vi "Unsubscribe.vi"(8 "error in (no error)":errorcluster, 10 "Message In":refnum<class "Message.lvclass">, 11 "System Actor in":refnum<class "System Actor.lvclass">) -> (0 "error out":errorcluster, 3 "System Actor out":refnum<class "System Actor.lvclass">)   [LabVIEW 2019, in "System Actor.lvclass"]
uses:
  System Actor.lvclass
  Message/Message.lvclass
  Message/Message.lvclass/Message.ctl
  System Actor.lvclass/System Actor.ctl
  Message/Public Data/Read Subscriber.vi
  Subscriber/Subscriber.lvclass
  Observer/Observer.lvclass
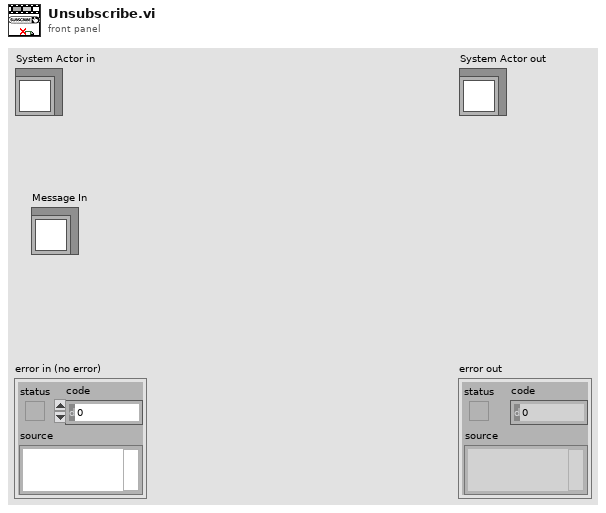
[diagram p1: front panel]
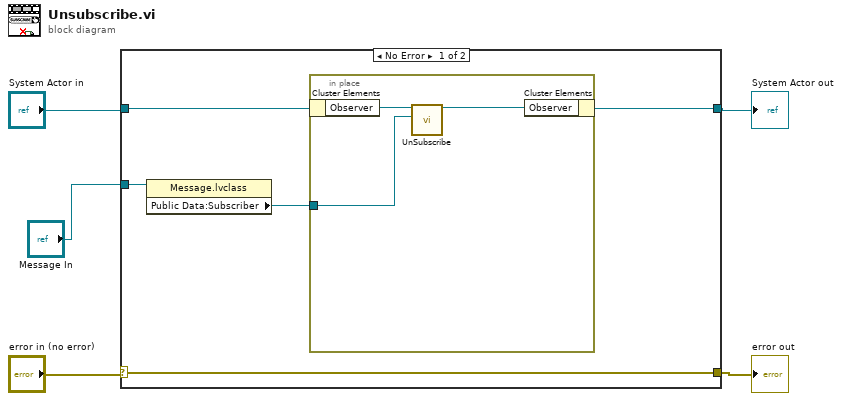
[diagram p0: block diagram]
diagram:
  n1 = case shown="No Error" "error in (no error)" {
    selector: "error in (no error)" -> [w10 w15]
    tunnel: [w10 w15] -> w1
    tunnel: [w7 w14] -> w2
    tunnel: "System Actor in" -> [w8 w14]
    tunnel: "Message In" -> [w9 _]
    frame No Error {
      n2 = property class="Message.lvclass"(reference=w9) -> ("Public Data:Subscriber"=w6:refnum<class "Subscriber.lvclass">)  [unwired: 1 in, 2 out]
      n3 = in-place {
        in-place-border: w6 -> [w11]
        n4 = in-place-cluster #1(w8) -> ("Observer"=w13:refnum<class "Observer.lvclass">)
        n5 = call-dynamic "UnSubscribe.vi"("Subscriber In"=w11, "Observer in"=w13) -> ("Observer out"=w12:refnum<class "Observer.lvclass">)  [unwired: 8 in, 1 out]
        n6 = in-place-cluster #1("Observer"=w12) -> (w7:refnum<class "System Actor.lvclass">)
      }
    }
    frame Error {
    }
  }
  "error out" <- w1
  "System Actor out" <- w2
